vi "Set Message obj.vi"(8 "error in (no error)":errorcluster caption="entrée d'erreur (pas d'erreur)", 9 "Message type":T1="Control", 10 "Message.lvclass":refnum<class "Message.lvclass">, 11 "Detector en entrée":refnum<class "Detector.lvclass">) -> (0 "error out":errorcluster caption="sortie d'erreur", 3 "Detector en sortie":refnum<class "Detector.lvclass">)   [LabVIEW 2015]
uses:
  Detector.lvclass
  Message/Message.lvclass
  dependecies/ControlsVIs/Clusters-def/Message types.ctl
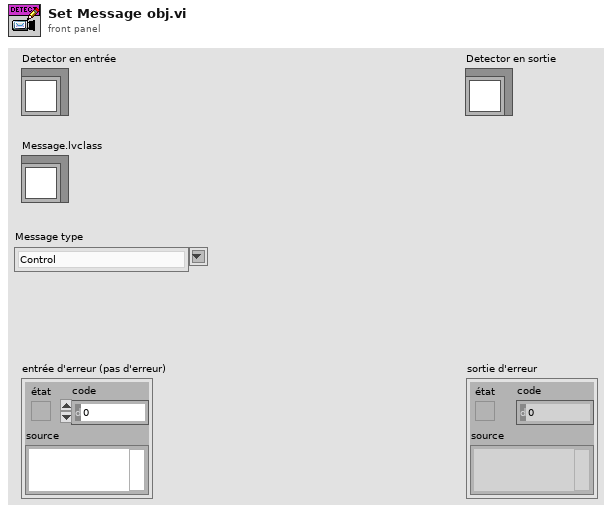
[diagram p1: front panel]
types:
  T1 = typedef "Message types.ctl" = string
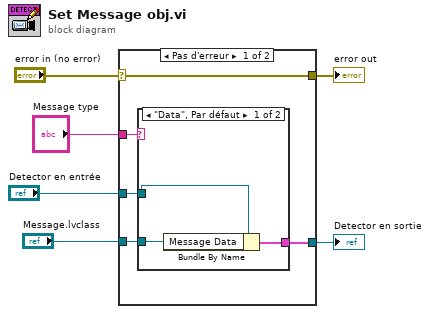
[diagram p0: block diagram]
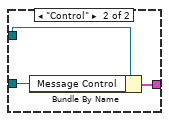
[diagram p2: hidden frame]
diagram:
  n1 = case shown="Pas d'erreur" "error in (no error)" {
    selector: "error in (no error)" -> [w11 w18]
    tunnel: [w11 w18] -> w5
    tunnel: [w9 w19] -> w3
    tunnel: "Detector en entrée" -> [w10 w19]
    tunnel: "Message.lvclass" -> [w8 _]
    tunnel: "Message type" -> [w7 _]
    frame No Error {
      n2 = case shown="\"Data\", Par défaut" w7 {
        tunnel: w10 -> [w14 w17]
        tunnel: [w13 w16] -> w9
        tunnel: w8 -> [w12 w15]
        frame "Data", Default {
          n3 = Bundle By Name(cluster=w14, "Message Data"=w12) -> (w13:cluster{})
        }
        frame "Control" {
          n4 = Bundle By Name(cluster=w17, "Message Control"=w15) -> (w16:cluster{})
        }
      }
    }
    frame Error {
    }
  }
  "error out" <- w5
  "Detector en sortie" <- w3
